vi "Get current pH.vi"(7 "beep (off)":bool, 8 "previous values":T1 {"time (s)" format="%.2f"; "temperature" format="%.2f"; "channel 2" format="%.2f"; "channel 1" format="%.2f"}, 9 "seconds/data point":u16, 10 "2nd channel":bool, 11 "Serial Port":enum16{"Modem port ", "Printer port"}(ring)) -> (0 "current values":T1 {"time (s)" format="%.2f"; "temperature" format="%.2f"; "channel 2" format="%.3f"; "channel 1" format="%.3f"}, 1 "units B":string, 2 "units A":string, 3 "Sample ID":u16, 5 "got data":bool)   [LabVIEW 2010]
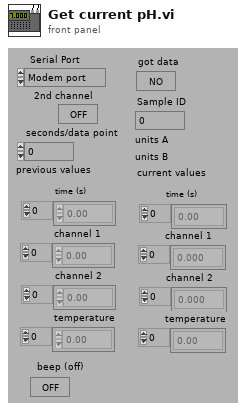
[diagram p1: front panel]
types:
  T1 = cluster{"channel 1":dbl[], "channel 2":dbl[], "temperature":dbl[], "time (s)":sgl[]}
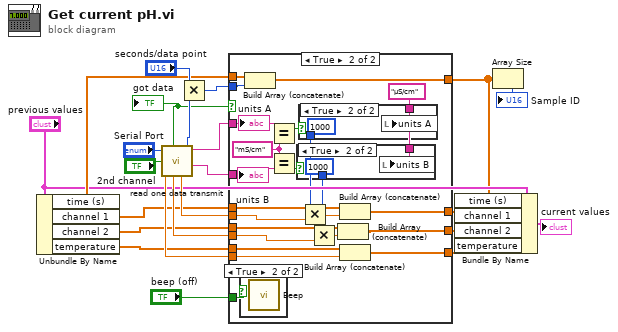
[diagram p0: block diagram]
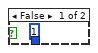
[diagram p3: hidden frame]
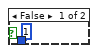
[diagram p4: hidden frame]
diagram:
  n1 = Unbundle By Name("previous values") -> ("time (s)"=w12:sgl[], "channel 1"=w11:dbl[], "channel 2"=w10:dbl[], "temperature"=w9:dbl[])
  n2 = call "read one data transmit.vi"("Serial Port"="Serial Port", "2nd channel"="2nd channel") -> ("got data"=w1:bool, "Temperature"=w14:sgl, "Channel 2"=w22:sgl, "Sample ID"=w18:u32, "Channel 1 units"=w20:string, "Channel 1"=w23:sgl, "Channel 2 units"=w19:string)  [unwired: 2 out]
  "got data" <- w1
  n3 = Multiply(x="seconds/data point", y=w18) -> (x*y=w21:u32)
  n4 = case shown="True" w1 {
    tunnel: [w25 w50] -> w3
    tunnel: [w26 w49] -> w4
    tunnel: [w27 w48] -> w5
    tunnel: w9 -> [w25 w47]
    tunnel: w10 -> [w26 w46]
    tunnel: w11 -> [w27 w45]
    tunnel: w14 -> [_ w44]
    tunnel: w22 -> [_ w43]
    tunnel: w23 -> [_ w42]
    tunnel: w12 -> [w24 w41]
    tunnel: [w24 w40] -> w6
    tunnel: w21 -> [_ w39]
    tunnel: w20 -> [_ w38]
    tunnel: w19 -> [_ w35]
    tunnel: "beep (off)" -> [_ w37]
    frame False {
    }
    frame True {
      w28 = "µS/cm"
      w36 = "mS/cm"
      n5 = case shown="True" w37 {
        frame False {
        }
        frame True {
          n6 = call <vilib>:"Beep.vi"() -> ()  [unwired: 12 in]
        }
      }
      n7 = Build Array (concatenate)(w41, w39) -> (w40:sgl[])
      n8 = Equal?(x=w38, y=w36) -> (x = y?=w34:bool)
      n9 = Equal?(x=w36, y=w35) -> (x = y?=w31:bool)
      n10 = case shown="True" w31 {
        tunnel: [1 1000] -> w29
        tunnel: w28 -> [_ w52]
        frame False {
        }
        frame True {
          n11 = local write "units B"(w52) -> ()
        }
      }
      n12 = case shown="True" w34 {
        tunnel: [1 1000] -> w32
        tunnel: w28 -> [_ w55]
        frame False {
        }
        frame True {
          n13 = local write "units A"(w55) -> ()
        }
      }
      n14 = Multiply(x=w32, y=w42) -> (x*y=w33:sgl)
      n15 = Multiply(x=w29, y=w43) -> (x*y=w30:sgl)
      n16 = Build Array (concatenate)(w46, w30) -> (w49:dbl[])
      n17 = Build Array (concatenate)(w45, w33) -> (w48:dbl[])
      n18 = Build Array (concatenate)(w47, w44) -> (w50:dbl[])
      "units B" <- w35
      "units A" <- w38
    }
  }
  n19 = Bundle By Name(cluster="previous values", "time (s)"=w6, "channel 1"=w5, "channel 2"=w4, "temperature"=w3) -> (→"current values":T1)
  n20 = Array Size(array=w6) -> (size(s)=→"Sample ID":i32)
